vi "Get Base messages for commands (SubVI).vi"(10 "result string in":string, 11 "ID":string) -> (2 "result string out":string, 3 "Communication out":T1 {"DATA[0]" format="%.0x"; "DATA[1]" format="%.0x"; "DATA[2]" format="%.0x"; "DATA[3]" format="%.0x"; "DATA[4]" format="%.0x"; "DATA[5]" format="%.0x"; "DATA[6]" format="%.0x"; "DATA[7]" format="%.0x"})   [LabVIEW 2025]
panel:
  out "error out":errorcluster
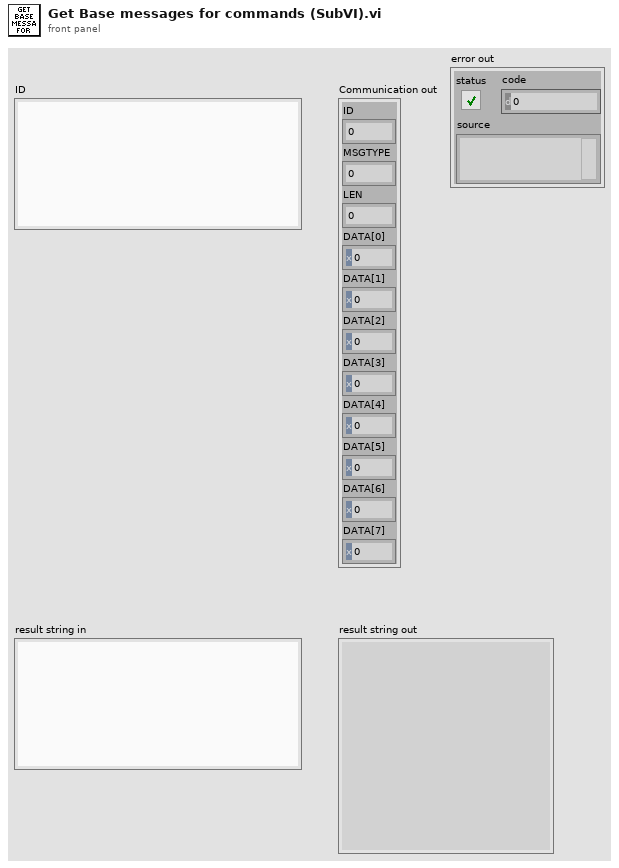
[diagram p1: front panel]
types:
  T1 = cluster{"ID":u32, "MSGTYPE":u8, "LEN":u8, "DATA[0]":u8, "DATA[1]":u8, "DATA[2]":u8, "DATA[3]":u8, "DATA[4]":u8, "DATA[5]":u8, "DATA[6]":u8, "DATA[7]":u8}
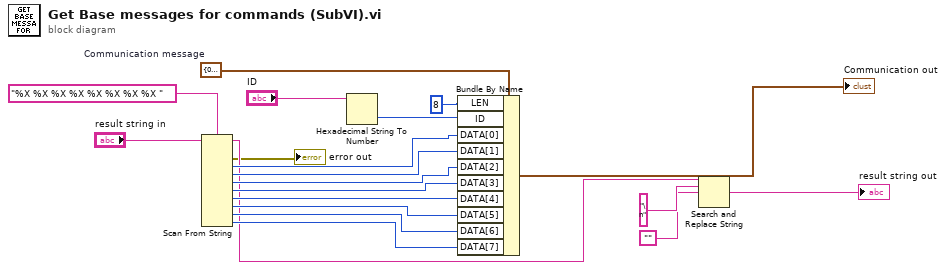
[diagram p0: block diagram]
diagram:
  w20 = T1 {"ID"=0, "MSGTYPE"=0, "LEN"=0, "DATA[0]"=0, "DATA[1]"=0, "DATA[2]"=0, "DATA[3]"=0, "DATA[4]"=0, "DATA[5]"=0, "DATA[6]"=0, "DATA[7]"=0}  # Communication message
  n1 = Scan From String(format string="%X %X %X %X %X %X %X %X ", input string="result string in") -> (remaining string=w7:string, error out=→"error out":errorcluster, output 1=w16:u32, output 2=w17:u32, output 3=w15:u32, output 4=w14:u32, output 5=w13:u32, output 6=w12:u32, output 7=w11:u32, output 8=w10:u32)  [unwired: 10 in, 1 out]
  n2 = Hexadecimal String To Number(string="ID") -> (number=w3:u32)  [unwired: 2 in, 1 out]
  n3 = Bundle By Name(cluster=w20, "LEN"=u8 8, "ID"=w3, "DATA[0]"=w16, "DATA[1]"=w17, "DATA[2]"=w15, "DATA[3]"=w14, "DATA[4]"=w13, "DATA[5]"=w12, "DATA[6]"=w11, "DATA[7]"=w10) -> (→"Communication out":T1)
  n4 = Search and Replace String(input string=w7, search string="\n", replace string="") -> (result string=→"result string out":string)  [unwired: 5 in, 3 out]
